vi "Excersie_4.vi"() -> ()   [LabVIEW 2013]
uses:
  <vilib>/Analysis/baseanly.llb/Mean (DBL).vi
  <vilib>/Analysis/NI_AALBase.lvlib
panel:
  in  "Thermometer":dbl(slide) scale=0.0..100.0
  out "Thermometer value":dbl
  in  "stop":bool
  out "mean":dbl format="%0.2f"
  out "max value":dbl
  out "min value":dbl
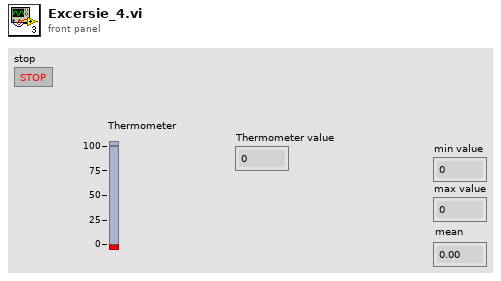
[diagram p1: front panel]
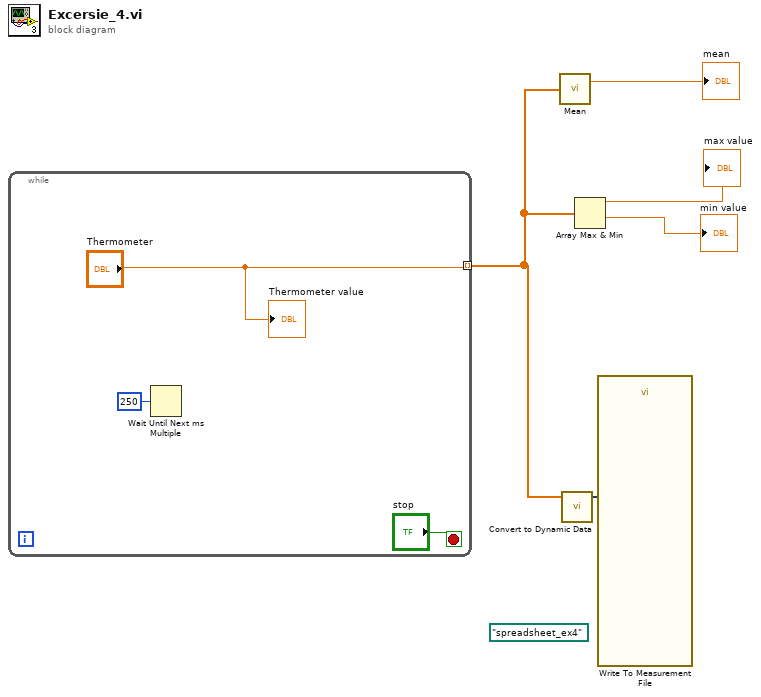
[diagram p0: block diagram]
diagram:
  (unwired) path "spreadsheet_ex4" ("Filename Out")
  n1 = while {
    tunnel: ["Thermometer"] -> w2 mode=indexing
    stop <- "stop" stop-if-true
    n2 = Wait Until Next ms Multiple(millisecond multiple=u32 250) -> ()  [unwired: 1 out]
    "Thermometer value" <- "Thermometer"
  }
  n3 = call-poly <vilib>:"Mean.vi"("X"=w2) -> ("mean"=→"mean":dbl)  [unwired: 1 out]
  n4 = call "Convert to Dynamic Data"("Array"=w2) -> ("Dynamic Data Type"=w1:dynamicdata)  [unwired: 3 in]
  n5 = Array Max & Min(array=w2) -> (max value=→"max value":dbl, min value=→"min value":dbl)  [unwired: 2 out]
  n6 = call "Write To Measurement File"("Signals"=w1) -> ()  [unwired: 16 in, 3 out]
